vi "concatenacion_señal_temperatura.vi"() -> ()   [LabVIEW 2020]
panel:
  in  "Slide":dbl(slide) scale=0.0..100.0
  in  "stop":bool
  out "Boolean":bool
  out "Waveform Chart":dynamicdata(graph)
  in  "Numeric":dbl
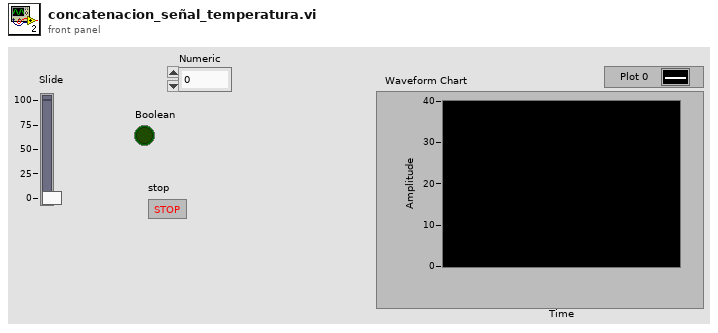
[diagram p1: front panel]
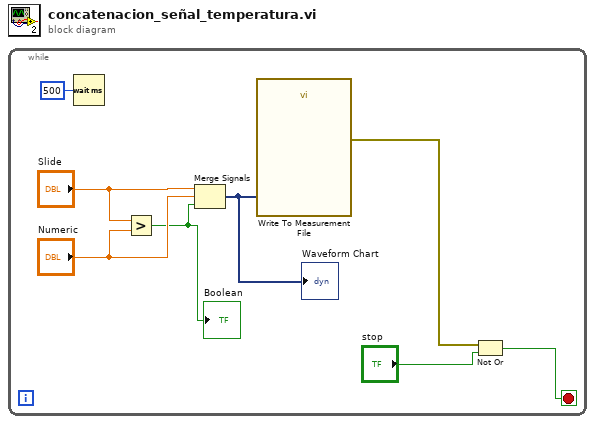
[diagram p0: block diagram]
diagram:
  n1 = while {
    stop <- w5 stop-if-true
    n2 = Wait (ms)(milliseconds to wait=u32 500) -> ()  [unwired: 1 out]
    n3 = Greater?(x="Slide", y="Numeric") -> (0:w2:bool)
    "Boolean" <- w2
    n4 = Merge Signals("Slide", "Numeric", w2) -> (w1:dynamicdata)
    "Waveform Chart" <- w1
    n5 = call "Write To Measurement File"("Signals"=w1) -> ("error out"=w7:errorcluster)  [unwired: 16 in, 2 out]
    n6 = Not Or(1:"stop", 2:w7) -> (0:w5:bool)
  }
